vi "Destroy.vi"(0 "reference":refnum<class "ClassNode.lvclass">, 5 "error in (no error)":errorcluster) -> (14 "reference out":refnum<class "ClassNode.lvclass">, 19 "error out":errorcluster)   [LabVIEW 2016, in "ClassNode.lvclass"]
doc: "Destroys a ClassNode object created with a ClassNode constructor VI.\n\n[GOOP 2.1]"
uses:
  <resource>/Framework/Providers/Open_GDS/UML/ClassNode_class/ClassNode.lvclass
  <resource>/Framework/Providers/Open_GDS/UML/RectangularNode_class/RectangularNode.lvclass
  <resource>/Framework/Providers/Open_GDS/UML/MultiLineString_class/MultiLineString.lvclass
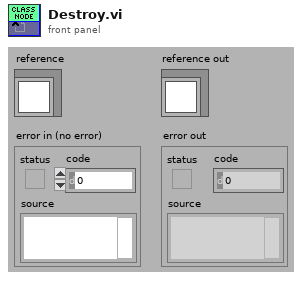
[diagram p1: front panel]
types:
  T1 = typedef "ClassNode.lvclass/ObjectAttributes.ctl" = cluster{"midHeight":dbl, "botHeight":dbl, "name":refnum<class "MultiLineString.lvclass">, "attributes":refnum<class "MultiLineString.lvclass">, "methods":refnum<class "MultiLineString.lvclass">, "DEFAULT_COMPARTMENT_HEIGHT":i32, "DEFAULT_WIDTH":i32, "DEFAULT_HEIGHT":i32, "showMethods":bool, "showAttributes":bool, "ClassPath":path}
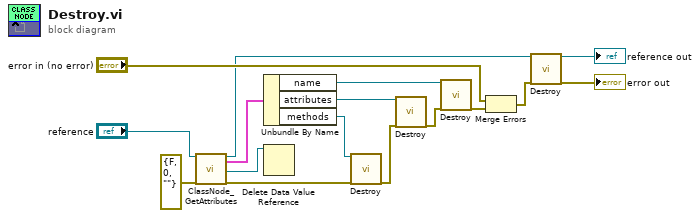
[diagram p0: block diagram]
diagram:
  n1 = call <resource>:"ClassNode_GetAttributes.vi"("reference in"="reference", "error in (no error)"=errorcluster {"status"=FALSE, "code"=0, "source"=""}) -> ("reference out"=w5:refnum<class "ClassNode.lvclass">, "Data"=w3:T1, "DataRef"=w2:refnum<data-value>, "error out"=w9:errorcluster)  [unwired: 1 in, 13 out]
  n2 = Unbundle By Name(w3) -> ("name"=w10:refnum<class "MultiLineString.lvclass">, "attributes"=w11:refnum<class "MultiLineString.lvclass">, "methods"=w12:refnum<class "MultiLineString.lvclass">)
  n3 = Delete Data Value Reference(data value reference=w2) -> ()  [unwired: 1 in, 2 out]
  n4 = call-dynamic "Destroy.vi"("reference"=w12, "error in (no error)"=w9) -> ("error out"=w8:errorcluster)  [unwired: 16 in, 1 out]
  n5 = call-dynamic "Destroy.vi"("reference"=w11, "error in (no error)"=w8) -> ("error out"=w7:errorcluster)  [unwired: 16 in, 1 out]
  n6 = call-dynamic "Destroy.vi"("reference"=w10, "error in (no error)"=w7) -> ("error out"=w6:errorcluster)  [unwired: 16 in, 1 out]
  n7 = Merge Errors("error in (no error)", w6) -> (w4:errorcluster)
  n8 = call-parent "Destroy.vi"("reference"=w5, "error in (no error)"=w4) -> ("reference out"=→"reference out":refnum<class "ClassNode.lvclass">, "error out"=→"error out":errorcluster)  [unwired: 16 in]
